vi "Mit Funktionstasten in STBY.vi"(11 "ausgewählte Funktion":T1) -> ()   [LabVIEW 2015]
uses:
  Funktionstasten/Funktionstasten.lvlib
  Aktion STY_MES.ctl
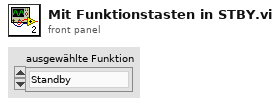
[diagram p1: front panel]
types:
  T1 = typedef "Funktionstasten.lvlib/Zustände.ctl" = enum16{"Standby", "Pause", "Eco", "Messen", "Kalibrieren", "Filter spülen", "Leitung spülen", "Umgebungsluft", "0-Gas", "Cal-Gas 1", "-------------", "Init 1", "Init 2", "Init 3", "Init 4", "Messen vorbereiten", "Messen durchführen", "Exit"}
  T2 = typedef "FID.lvlib/Aktion STY_MES.ctl" = enum16{"lesen", "setze STY", "setze MES", "MODBUS schreiben"}
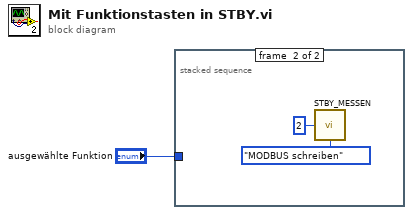
[diagram p0: block diagram]
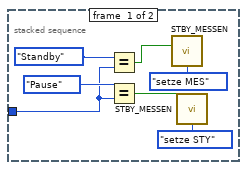
[diagram p2: hidden frame]
diagram:
  n1 = stacked-sequence {
    tunnel: "ausgewählte Funktion" -> [w2 _]
    frame #0 {
      n2 = Equal?(x=Zustände."Standby", y=w2) -> (x = y?=w5:bool)
      n3 = Equal?(x=Zustände."Pause", y=w2) -> (x = y?=w3:bool)
      n4 = call "STBY_MESSEN.vi"("Messen"=w5, "Aktion"=Aktion_STY_MES."setze MES") -> ()  [unwired: 10 in, 4 out]
      n5 = call "STBY_MESSEN.vi"("Standby"=w3, "Aktion"=Aktion_STY_MES."setze STY") -> ()  [unwired: 10 in, 4 out]
    }
    frame #1 {
      n6 = call "STBY_MESSEN.vi"("Case Nr."=2, "Aktion"=Aktion_STY_MES."MODBUS schreiben") -> ()  [unwired: 10 in, 4 out]
    }
  }
